vi "Scan action control via Global Variables.vi"(0 "Index":i32, 1 "OSC Configuration":T2(array[cluster])=[{"Signal Type"=enum."Sawtooth Wave", "DC"=0.00055, "Amplitude"=0.002, "frequency"=0.25, "Phase"=180.0}, {"Signal Type"=enum."Sine Wave", "DC"=0.0, "Amplitude"=0.0, "frequency"=1.0, "Phase"=0.0}, {"Signal Type"=enum."Sine Wave", "DC"=0.0, "Amplitude"=0.0, "frequency"=1.0, "Phase"=0.0}, {"Signal Type"=enum."Sine Wave", "DC"=0.0, "Amplitude"=0.0, "frequency"=1.0, "Phase"=0.0}] {"frequency" format="%0.2p"; "Amplitude" format="%0.2p"; "DC" format="%.2p"}, 2 "Scan control":u16(ring)=1 items=["OFF", "Vsg1", "Vsg2", "Vsgw", "Vbg", "Field", "Temp", "Position"], 3 "Scan Parameters":T1={"DAQ Channel"=2, "Label"="\nscaledVsg1=", "Scaled low"=-0.060000000000000005, "Scaled high"=0.14, "Start"=0.14, "End"=-0.060000000000000005, "Step"=-0.060000000000000005, "Scale?"=TRUE} {"Step" format="%#_6p"; "End" format="%#_6p"; "Start" format="%#_6p"; "Scaled high" format="%#_6p"; "Scaled low" format="%#_6p"}, 4 "Comments":string) -> (5 "Comments out":string, 6 "OSC Configuration out":T2(array[cluster])=[{"Signal Type"=enum."Sawtooth Wave", "DC"=0.00055, "Amplitude"=0.002, "frequency"=0.25, "Phase"=180.0}, {"Signal Type"=enum."Sine Wave", "DC"=0.0, "Amplitude"=0.0, "frequency"=1.0, "Phase"=0.0}, {"Signal Type"=enum."Sine Wave", "DC"=0.0, "Amplitude"=0.0, "frequency"=1.0, "Phase"=0.0}, {"Signal Type"=enum."Sine Wave", "DC"=0.0, "Amplitude"=0.0, "frequency"=1.0, "Phase"=0.0}] {"frequency" format="%0.2p"; "Amplitude" format="%0.2p"; "DC" format="%.2p"}, 7 "Stop?":bool)   [LabVIEW 2013]
panel:
  in  "Rate (K/min)":dbl=5.0
  in  "Rate (Oe/s)":i32=30
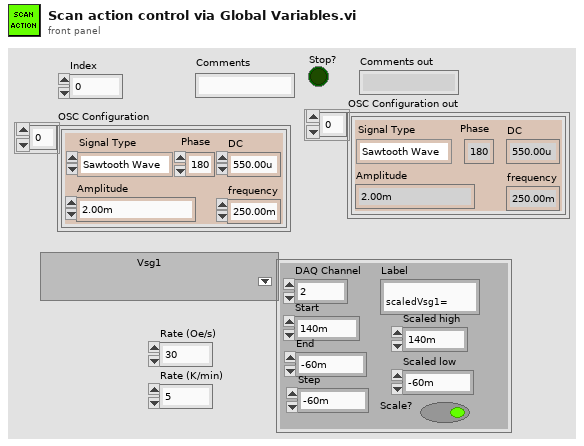
[diagram p1: front panel]
types:
  T1 = cluster{"DAQ Channel":i32, "Label":string, "Scaled low":dbl, "Scaled high":dbl, "Start":dbl, "End":dbl, "Step":dbl, "Scale?":bool}
  T2 = cluster{"Signal Type":enum16{"Sine Wave", "Triangle Wave", "Square Wave", "Sawtooth Wave"}, "DC":dbl, "Amplitude":dbl, "frequency":dbl, "Phase":dbl}[]
  T3 = cluster{"Signal Type":enum16{"Sine Wave", "Triangle Wave", "Square Wave", "Sawtooth Wave"}, "DC":dbl, "Amplitude":dbl, "frequency":dbl, "Phase":dbl}
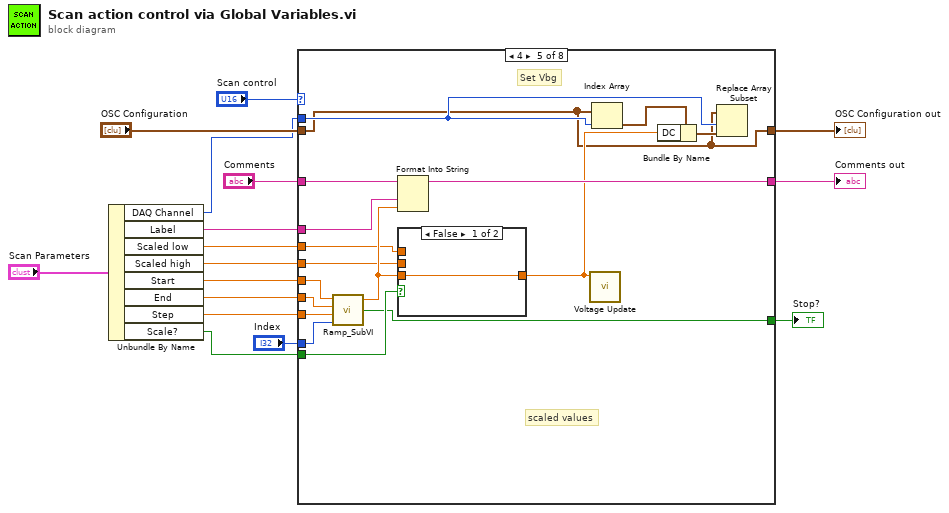
[diagram p0: block diagram]
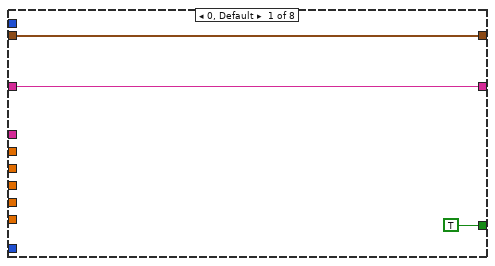
[diagram p2: hidden frame]
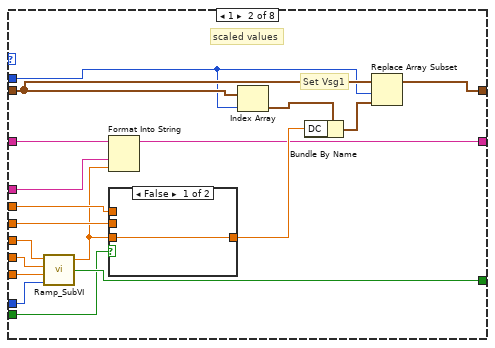
[diagram p3: hidden frame]
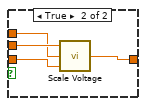
[diagram p4: hidden frame]
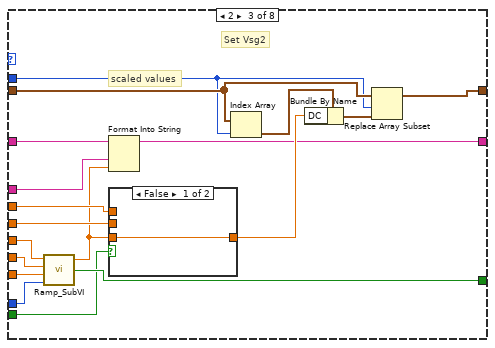
[diagram p5: hidden frame]
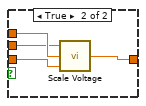
[diagram p6: hidden frame]
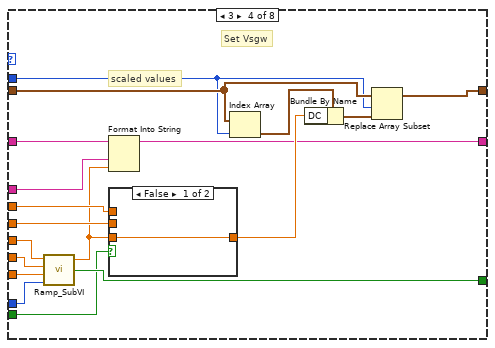
[diagram p7: hidden frame]
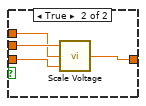
[diagram p8: hidden frame]
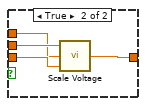
[diagram p9: hidden frame]
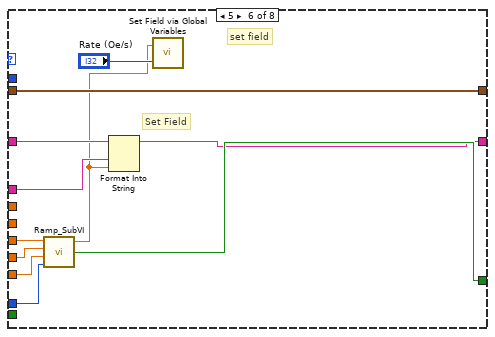
[diagram p10: hidden frame]
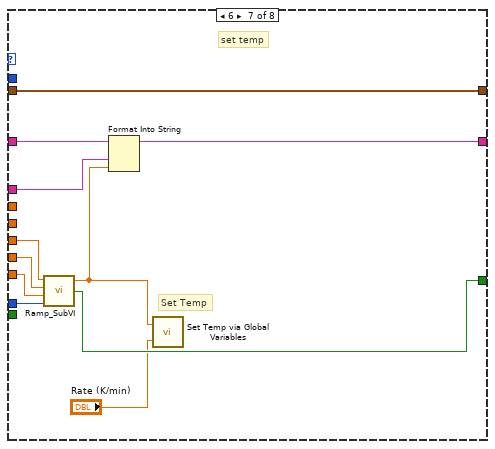
[diagram p11: hidden frame]
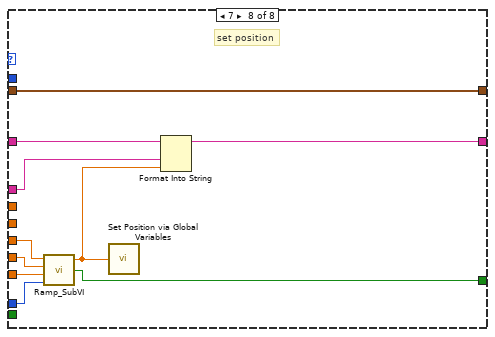
[diagram p12: hidden frame]
diagram:
  n1 = Unbundle By Name("Scan Parameters") -> ("DAQ Channel"=w1:i32, "Label"=w13:string, "Scaled low"=w4:dbl, "Scaled high"=w3:dbl, "Start"=w8:dbl, "End"=w7:dbl, "Step"=w6:dbl, "Scale?"=w2:bool)
  n2 = case shown="4" "Scan control" {
    tunnel: "OSC Configuration" -> [w19 w36 w59 w82 w89 w121 w132 w142]
    tunnel: w1 -> [_ w35 w58 w81 w98 _ _ _]
    tunnel: [w19 w33 w56 w79 w89 w121 w132 w142] -> w12
    tunnel: "Comments" -> [w18 w21 w46 w67 w99 w115 w125 w139]
    tunnel: [w18 w22 w43 w68 w92 w113 w124 w135] -> w11
    tunnel: w13 -> [_ w20 w45 w66 w97 w114 w126 w140]
    tunnel: "Index" -> [_ w32 w55 w78 w101 w120 w128 w137]
    tunnel: w8 -> [_ w31 w54 w77 w93 w119 w131 w141]
    tunnel: w7 -> [_ w30 w53 w76 w94 w118 w130 w134]
    tunnel: w6 -> [_ w29 w52 w75 w100 w117 w129 w138]
    tunnel: [TRUE ("Stop?") w28 w51 w74 w91 w116 w127 w133] -> w5
    tunnel: w4 -> [_ w26 w50 w72 w95 _ _ _]
    tunnel: w3 -> [_ w27 w49 w73 w96 _ _ _]
    tunnel: w2 -> [_ w24 w47 w70 w102 _ _ _]
    frame 0, Default {
    }
    frame 1 {
      # "Set Vsg1"
      # "scaled values"
      n3 = call <userlib>:"Ramp_SubVI.vi"("index"=w32, "step"=w29, "end"=w30, "start"=w31) -> ("Stop?"=w28:bool, "Numeric"=w23:dbl)  [unwired: 1 in]
      n4 = Format Into String(initial string=w21, w20, w23) -> (resulting string=w22:string)  [unwired: 2 in, 1 out]
      n5 = case shown="False" w24 {
        tunnel: w27 -> [_ w42]
        tunnel: w26 -> [_ w41]
        tunnel: w23 -> [w38 w40]
        tunnel: [w38 w39] -> w25
        frame False {
        }
        frame True {
          n6 = call <userlib>:"Scale Voltage.vi"("Scale factor"=w40, "Breakdown Low"=w41, "Breakdown High"=w42) -> ("Real Voltage"=w39:dbl)
        }
      }
      n7 = Index Array(array=w36, index=w35) -> (element=w37:T3)
      n8 = Bundle By Name(cluster=w37, "DC"=w25) -> (w34:T3)
      n9 = Replace Array Subset(array=w36, new element=w34, index=w35) -> (w33:T2)
    }
    frame 2 {
      # "Set Vsg2"
      # "scaled values"
      n10 = call <userlib>:"Ramp_SubVI.vi"("index"=w55, "step"=w52, "end"=w53, "start"=w54) -> ("Stop?"=w51:bool, "Numeric"=w44:dbl)  [unwired: 1 in]
      n11 = Format Into String(initial string=w46, w45, w44) -> (resulting string=w43:string)  [unwired: 2 in, 1 out]
      n12 = case shown="False" w47 {
        tunnel: w50 -> [_ w65]
        tunnel: w49 -> [_ w64]
        tunnel: w44 -> [w61 w63]
        tunnel: [w61 w62] -> w48
        frame False {
        }
        frame True {
          n13 = call <userlib>:"Scale Voltage.vi"("Scale factor"=w63, "Breakdown Low"=w65, "Breakdown High"=w64) -> ("Real Voltage"=w62:dbl)
        }
      }
      n14 = Index Array(array=w59, index=w58) -> (element=w60:T3)
      n15 = Bundle By Name(cluster=w60, "DC"=w48) -> (w57:T3)
      n16 = Replace Array Subset(array=w59, new element=w57, index=w58) -> (w56:T2)
    }
    frame 3 {
      # "Set Vsgw"
      # "scaled values"
      n17 = call <userlib>:"Ramp_SubVI.vi"("index"=w78, "step"=w75, "end"=w76, "start"=w77) -> ("Stop?"=w74:bool, "Numeric"=w69:dbl)  [unwired: 1 in]
      n18 = Format Into String(initial string=w67, w66, w69) -> (resulting string=w68:string)  [unwired: 2 in, 1 out]
      n19 = case shown="False" w70 {
        tunnel: w69 -> [w84 w88]
        tunnel: w73 -> [_ w87]
        tunnel: w72 -> [_ w86]
        tunnel: [w84 w85] -> w71
        frame False {
        }
        frame True {
          n20 = call <userlib>:"Scale Voltage.vi"("Scale factor"=w88, "Breakdown Low"=w86, "Breakdown High"=w87) -> ("Real Voltage"=w85:dbl)
        }
      }
      n21 = Index Array(array=w82, index=w81) -> (element=w83:T3)
      n22 = Bundle By Name(cluster=w83, "DC"=w71) -> (w80:T3)
      n23 = Replace Array Subset(array=w82, new element=w80, index=w81) -> (w79:T2)
    }
    frame 4 {
      # "Set Vbg"
      # "scaled values"
      n24 = call <userlib>:"Ramp_SubVI.vi"("index"=w101, "step"=w100, "end"=w94, "start"=w93) -> ("Stop?"=w91:bool, "Numeric"=w103:dbl)  [unwired: 1 in]
      n25 = Format Into String(initial string=w99, w97, w103) -> (resulting string=w92:string)  [unwired: 2 in, 1 out]
      n26 = case shown="False" w102 {
        tunnel: w103 -> [w106 w110]
        tunnel: w96 -> [_ w109]
        tunnel: w95 -> [_ w108]
        tunnel: [w106 w107] -> w90
        frame False {
        }
        frame True {
          n27 = call <userlib>:"Scale Voltage.vi"("Scale factor"=w110, "Breakdown Low"=w108, "Breakdown High"=w109) -> ("Real Voltage"=w107:dbl)
        }
      }
      n28 = call "Voltage Update.vi"("Voltage Output (to Backgate)"=w90) -> ()  [unwired: 8 in]
      n29 = Index Array(array=w89, index=w98) -> (element=w105:T3)
      n30 = Bundle By Name(cluster=w105, "DC"=w90) -> (w104:T3)
      n31 = Replace Array Subset(array=w89, new element=w104, index=w98) -> ()  [unwired: 1 out]
    }
    frame 5 {
      # "Set Field"
      # "set field"
      n32 = call <userlib>:"Ramp_SubVI.vi"("index"=w120, "step"=w117, "end"=w118, "start"=w119) -> ("Stop?"=w116:bool, "Numeric"=w111:dbl)  [unwired: 1 in]
      n33 = Format Into String(initial string=w115, w114, w111) -> (resulting string=w113:string)  [unwired: 2 in, 1 out]
      n34 = call "Set Field via Global Variables.vi"("Rate (Oe/s)"="Rate (Oe/s)", "Field"=w111) -> ()  [unwired: 1 in]
    }
    frame 6 {
      # "Set Temp"
      # "set temp"
      n35 = call <userlib>:"Ramp_SubVI.vi"("index"=w128, "step"=w129, "end"=w130, "start"=w131) -> ("Stop?"=w127:bool, "Numeric"=w122:dbl)  [unwired: 1 in]
      n36 = Format Into String(initial string=w125, w126, w122) -> (resulting string=w124:string)  [unwired: 2 in, 1 out]
      n37 = call "Set Temp via Global Variables.vi"("Rate"="Rate (K/min)", "Temperature"=w122) -> ()  [unwired: 1 in]
    }
    frame 7 {
      # "set position"
      n38 = call <userlib>:"Ramp_SubVI.vi"("index"=w137, "step"=w138, "end"=w134, "start"=w141) -> ("Stop?"=w133:bool, "Numeric"=w136:dbl)  [unwired: 1 in]
      n39 = call "Set Position via Global Variables.vi"("Position"=w136) -> ()  [unwired: 1 in]
      n40 = Format Into String(initial string=w139, w140, w136) -> (resulting string=w135:string)  [unwired: 2 in, 1 out]
    }
  }
  "OSC Configuration out" <- w12
  "Comments out" <- w11
  "Stop?" <- w5
